vi "startList.vi"(8 "error in (no error)":errorcluster, 10 "Listbox":refnum<vi>, 11 "ExperimentRunner in":refnum<class "ExperimentRunner.lvclass">) -> (0 "error out":errorcluster, 2 "Listbox out":refnum<vi>, 3 "ExperimentRunner out":refnum<class "ExperimentRunner.lvclass">)   [LabVIEW 2009, in "Views.lvlib" / "ExperimentControl.lvlib" / "ExperimentRunner.lvclass"]
doc: "Adds the new Script path name to the Front End."
uses:
  ExperimentRunner.lvclass
  ExperimentRunner.lvclass/ExperimentRunner.ctl
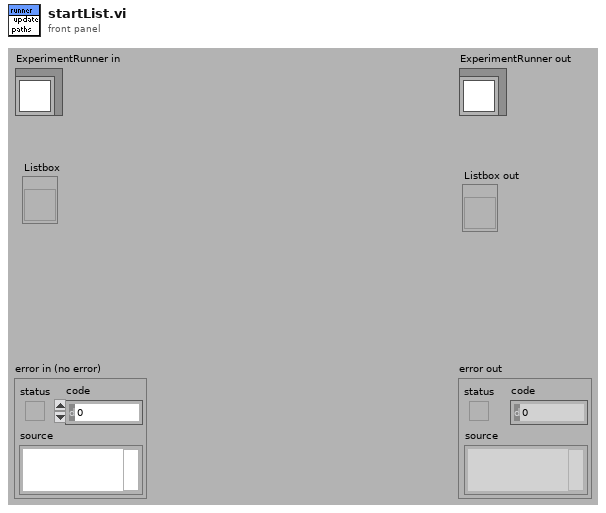
[diagram p1: front panel]
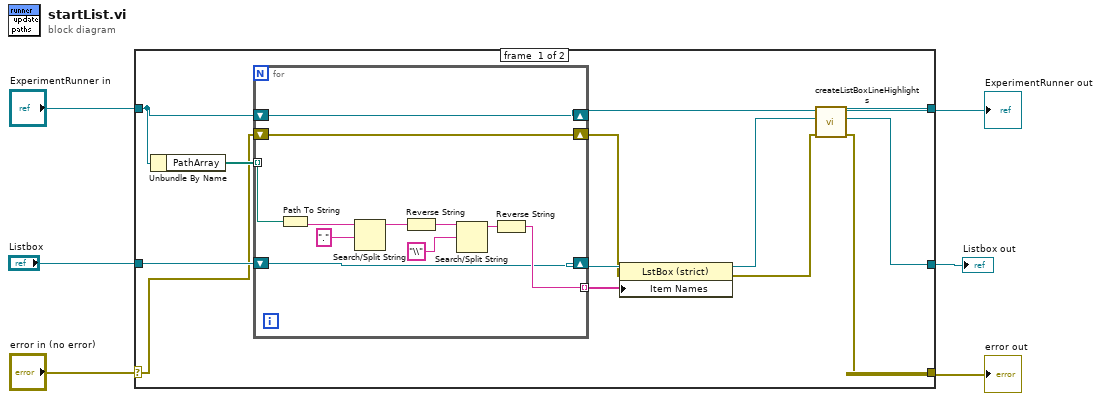
[diagram p0: block diagram]
diagram:
  n1 = case shown="No Error" "error in (no error)" {
    selector: "error in (no error)" -> [w9 w32]
    tunnel: [w15 w32] -> w5
    tunnel: [w14 w31] -> w3
    tunnel: "ExperimentRunner in" -> [w11 w31]
    tunnel: "Listbox" -> [w18 _]
    tunnel: [w12 _] -> w1
    frame #0 {
      n2 = Unbundle By Name(w11) -> ("PathArray"=w19:path[])
      n3 = for {
        tunnel: w19 -> [w24] mode=indexing
        shift-right: [w20] -> w17
        shift-left: w18 -> [w20]
        shift-right: [w23] -> w10
        shift-left: w11 -> [w23]
        shift-right: [w22] -> w8
        shift-left: w9 -> [w22]
        tunnel: [w21] -> w7 mode=indexing
        n4 = Path To String(path=w24) -> (string=w30:string)
        n5 = Search/Split String(string=w30, search string/char (-)=".") -> (substring before match=w28:string)  [unwired: 1 in, 2 out]
        n6 = Reverse String(1:w28) -> (0:w27:string)
        n7 = Search/Split String(string=w27, search string/char (-)="\\") -> (substring before match=w25:string)  [unwired: 1 in, 2 out]
        n8 = Reverse String(1:w25) -> (0:w21:string)
      }
      n9 = property class="LstBox (strict)"(reference=w17, error in=w8, "Item Names"=w7) -> (reference out=w13:refnum<vi>, error out=w16:errorcluster)
      n10 = call "createListBoxLineHighlights.vi"("error in (no error)"=w16, "Listbox in"=w13, "ExperimentRunner in"=w10) -> ("error out"=w15:errorcluster, "Listbox out"=w12:refnum<vi>, "ExperimentRunner out"=w14:refnum<class "ExperimentRunner.lvclass">)  [unwired: 6 in]
    }
    frame #1 {
    }
  }
  "error out" <- w5
  "ExperimentRunner out" <- w3
  "Listbox out" <- w1
